vi "UHR-Fleezers Control (host) - 11.9.vi"() -> ()   [LabVIEW 2014] (continued)
        n1091 = xnode "Read/Write Control"("FPGA VI Reference In"=w1467, "error in"=w1468, "+ phase (APD 2 Gate)"=w1465) -> ("error out"=w1466:errorcluster)  [unwired: 1 out]
      }
      event "Phase Adj. (APD Acq)", "+ phase (APD Acq)", "- phase (APD Acq)": Value Change {
        n1092 = event-data() -> ()  [unwired: 7 out]
        n1093 = local read "Phase Adj. (APD Acq)"() -> (w1475:i16)
        n1094 = Negate(x=w1475) -> (-x=w1481:i16)
        n1095 = Select(t=w1481, s="+ phase (APD Acq)", f=w1475) -> (s? t:f=w1480:i16)
        n1096 = Or(x="+ phase (APD Acq)", y="- phase (APD Acq)") -> (x .or. y?=w1476:bool)
        n1097 = xnode "Read/Write Control"("FPGA VI Reference In"=w1483, "error in"=w1482, "Phase Count Adjustment (APD Acq)"=w1480) -> ("FPGA VI Reference Out"=w1478:T19, "error out"=w1479:errorcluster)
        n1098 = xnode "Read/Write Control"("FPGA VI Reference In"=w1478, "error in"=w1479, "+ phase (APD Acq)"=w1476) -> ("error out"=w1477:errorcluster)  [unwired: 1 out]
      }
      event "Phase adj. (GI)", "+ phase (GI)", "- phase (GI)": Value Change {
        n1099 = event-data() -> ()  [unwired: 7 out]
        n1100 = Negate(x="Phase adj. (GI)") -> (-x=w1492:i16)
        n1101 = Select(t=w1492, s="+ phase (GI)", f="Phase adj. (GI)") -> (s? t:f=w1491:i16)
        n1102 = Or(x="+ phase (GI)", y="- phase (GI)") -> (x .or. y?=w1487:bool)
        n1103 = xnode "Read/Write Control"("FPGA VI Reference In"=w1494, "error in"=w1493, "Phase count adjustment (GI)"=w1491) -> ("FPGA VI Reference Out"=w1489:T19, "error out"=w1490:errorcluster)
        n1104 = xnode "Read/Write Control"("FPGA VI Reference In"=w1489, "error in"=w1490, "+ phase (GI)"=w1487) -> ("error out"=w1488:errorcluster)  [unwired: 1 out]
      }
      event "Phase adj. (GI) 2", "+ phase (GI) 2", "- phase (GI) 2": Value Change {
        n1105 = event-data() -> ()  [unwired: 7 out]
        n1106 = Negate(x="Phase adj. (GI) 2") -> (-x=w1503:i16)
        n1107 = Select(t=w1503, s="+ phase (GI) 2", f="Phase adj. (GI) 2") -> (s? t:f=w1502:i16)
        n1108 = Or(x="+ phase (GI) 2", y="- phase (GI) 2") -> (x .or. y?=w1498:bool)
        n1109 = xnode "Read/Write Control"("FPGA VI Reference In"=w1505, "error in"=w1504, "Phase count adjustment (GI) 2"=w1502) -> ("FPGA VI Reference Out"=w1500:T19, "error out"=w1501:errorcluster)
        n1110 = xnode "Read/Write Control"("FPGA VI Reference In"=w1500, "error in"=w1501, "+ phase (GI) 2"=w1498) -> ("error out"=w1499:errorcluster)  [unwired: 1 out]
      }
      event "Phase adj. (Green FB)", "- phase (Green FB)", "+ phase (Green FB)": Value Change {
        n1111 = event-data() -> ()  [unwired: 7 out]
        n1112 = Negate(x="Phase adj. (Green FB)") -> (-x=w1514:i16)
        n1113 = Select(t=w1514, s="+ phase (Green FB)", f="Phase adj. (Green FB)") -> (s? t:f=w1513:i16)
        n1114 = Or(x="+ phase (Green FB)", y="- phase (Green FB)") -> (x .or. y?=w1509:bool)
        n1115 = xnode "Read/Write Control"("FPGA VI Reference In"=w1516, "error in"=w1515, "Phase count adjustment (Green FB)"=w1513) -> ("FPGA VI Reference Out"=w1511:T19, "error out"=w1512:errorcluster)
        n1116 = xnode "Read/Write Control"("FPGA VI Reference In"=w1511, "error in"=w1512, "+ phase (Green FB)"=w1509) -> ("error out"=w1510:errorcluster)  [unwired: 1 out]
      }
      event "Invert APD Gate", "APD Gate ON Count", "APD Gate OFF Count", "APD Gate", "APD Integration Time (s)", "APD 1 AO Mult.", "APD 2 AO Mult.", "On one out of X cycles": Value Change {
        n1117 = event-data() -> ()  [unwired: 7 out]
        n1118 = Add(x="GI Frequency, ON count", y="GI Frequency, OFF count") -> (x+y=w1520:u32)
        n1119 = Add(x="APD Gate ON Count", y="APD Gate OFF Count") -> (x+y=w1533:u32)
        n1120 = Multiply(x="On one out of X cycles", y=w1520) -> (x*y=w1517:u32)
        "Green FB Count" <- w1517
        n1121 = Subtract(x=w1517, y="GI Frequency, ON count") -> (x-y=w1518:u32)
        n1122 = Multiply(x=w1533, y="On one out of X cycles") -> (x*y=w1532:u32)
        n1123 = Subtract(x=w1532, y="APD Gate ON Count") -> (x-y=w1531:u32)
        n1124 = local read "DMA Update Period (s)"() -> (w1534:dbl)
        n1125 = Multiply(x="APD Integration Time (s)", y=40000000.0) -> (x*y=w1539:dbl)
        n1126 = Reciprocal(x="APD Integration Time (s)") -> (1/x=→"APD Acq Rate (Hz)":dbl)
        n1127 = To Unsigned Long Integer(number=w1539) -> (unsigned 32bit integer=w1523:u32)
        "APD Int. Count" <- w1523
        n1128 = xnode "Read/Write Control"("FPGA VI Reference In"=w1543, "error in"=w1542, "Invert APD Gate"="Invert APD Gate", "APD Gate ON Count"="APD Gate ON Count", "APD Gate OFF Count"=w1531, "APD Acq Rate Count"=w1523, "APD Gate Operating Mode"="APD Gate", "APD 1 AO scale factor"="APD 1 AO Mult.", "APD 2 AO scale factor"="APD 2 AO Mult.", "Green interlace ON count"="GI Frequency, ON count", "Green interlace OFF count"=w1518, "Green interlace ON count 2"="GI Frequency, ON count", "Green interlace OFF count 2"=w1518, "Green FB Count"=w1517) -> ("error out"=w1541:errorcluster)  [unwired: 1 out]
        n1129 = Divide(x=w1534, y="APD Integration Time (s)") -> (x/y=w1537:dbl)
        n1130 = Multiply(x=2.0, y=w1537) -> (x*y=w1536:dbl)
        n1131 = local write "APD Samples/FIFO Acq."(w1537) -> ()
        n1132 = local write "APD Elements/DMA read"(w1536) -> ()
      }
      event "Number of F/B Scans (AOD)", "Scan Speed (nm/s)", "Scan BD", "Initial D (MHz)", "Step Size (nm)", "Scan Range (nm)", "Wiggle amp 1 (units?)": Value Change {
        w1605 = 123.0  # AOM cal (nm/MHz)
        n1133 = event-data() -> ()  [unwired: 7 out]
        n1134 = local read "BD 1 Frequency 1 (MHz)"() -> (w1588:dbl)
        n1135 = local read "AOM X Cal (nm/MHz)"() -> (w1580:dbl)
        n1136 = local read "BD 2 Frequency 1 (MHz)"() -> (w1594:dbl)
        n1137 = local read "X RF Frequency Limits (MHz)"() -> (w1592:T16)
        n1138 = local read "Y RF Frequency Limits (MHz)"() -> (w1589:T16)
        n1139 = Negate(x="Scan Range (nm)") -> (-x=w1558:dbl)
        n1140 = Divide(x=w1558, y=w1580) -> (x/y=w1562:dbl)
        n1141 = Select(t=w1592, s="Scan BD", f=w1589) -> (s? t:f=w1591:T16)
        n1142 = Select(t=w1588, s="Scan BD", f=w1594) -> (s? t:f=w1593:dbl)
        n1143 = Unbundle By Name(w1591) -> ("Maximum"=w1600:dbl, "Minimum"=w1599:dbl)
        n1144 = Add(x=w1562, y=w1593) -> (x+y=w1597:dbl)
        n1145 = Divide(x=w1558, y="Step Size (nm)") -> (x/y=w1577:dbl)
        n1146 = Divide(x="Step Size (nm)", y=w1580) -> (x/y=w1586:dbl)
        n1147 = Absolute Value(x=w1577) -> (abs(x)=w1561:dbl)
        n1148 = Sign(1:w1558) -> (0:w1559:dbl)
        n1149 = In Range and Coerce(upper limit=w1600, x=w1597, lower limit=w1599) -> (coerced(x)=w1596:dbl, In Range?=w1598:bool)
        n1150 = To Unsigned Quad Integer(1:w1561) -> (0:w1576:u64)
        "Scan steps (AOD)" <- w1576
        n1151 = call "IR AOM freq to word.vi"("Frequency In (MHz)"=w1586) -> ("Frequency Word Out (double)"=w1583:dbl)
        n1152 = Multiply(x=w1559, y=w1583) -> (x*y=w1560:dbl)
        n1153 = Subtract(x=w1597, y=w1596) -> (x-y=w1595:dbl)
        n1154 = To Quad Integer(1:w1560) -> (0:w1582:i64)
        "Incr. int (AOD)" <- w1582
        n1155 = Subtract(x=w1562, y=w1595) -> (x-y=w1581:dbl)
        "Scan Range (MHz)" <- w1581
        n1156 = Select(t=w1562, s=w1598, f=w1581) -> (s? t:f=w1601:dbl)
        n1157 = Multiply(x=w1581, y=w1580) -> (x*y=w1579:dbl)
        n1158 = Decrement(x=w1576) -> (x-1=w1629:u64)
        n1159 = Negate(x=w1579) -> (-x=w1575:dbl)
        n1160 = local write "Scan Range (nm)"(w1575) -> ()
        n1161 = Divide(x=w1601, y=w1629) -> (x/y=w1585:dbl)
        "Scan Increment (MHz)" <- w1585
        n1162 = call "IR AOM freq to word.vi"("Frequency In (MHz)"=w1585) -> ("Frequency Word Out (double)"=w1584:dbl)
        n1163 = Divide(x="Step Size (nm)", y="Scan Speed (nm/s)") -> (x/y=w1572:dbl)
        n1164 = To Quad Integer(1:w1584) -> ()  [unwired: 1 out]
        n1165 = local read "Number Interlace Sets"() -> (w1556:u8)
        n1166 = local read "AI Count (ticks)"() -> (w1557:u32)
        n1167 = local read "Total Counts (ticks)"() -> (w1555:u32)
        n1168 = local read "# Samples/trap"() -> (w1587:u32)
        n1169 = Multiply(x=w1557, y=w1556) -> (x*y=w1554:u32)
        n1170 = Divide(x=w1555, y=w1554) -> (x/y=w1553:dbl)
        n1171 = Select(t=w1588, s="Scan BD", f=w1594) -> (s? t:f=w1626:dbl)
        "Initial freq. (MHz)" <- w1626
        n1172 = Add(x=w1601, y=w1626) -> (x+y=→"Final freq. (MHz)":dbl)
        n1173 = Divide(x=w1555, y=40000000.0) -> (x/y=w1571:dbl)
        n1174 = Divide(x=w1572, y=w1571) -> (x/y=w1570:dbl)
        n1175 = To Unsigned Quad Integer(1:w1570) -> (0:w1545:u64)
        n1176 = Quotient & Remainder(x=w1545, y=u64 2) -> (x-y*floor(x/y)=w1549:u64)  [unwired: 1 out]
        n1177 = Equal?(x=w1549, y=u64 0) -> (x = y?=w1547:bool)
        n1178 = Decrement(x=w1545) -> (x-1=w1546:u64)
        n1179 = Select(t=w1545, s=w1547, f=w1546) -> (s? t:f=w1544:u64)
        "Cycles/step (AOD)" <- w1544
        n1180 = xnode "Read/Write Control"("FPGA VI Reference In"=w1637, "error in"=w1636, "Scan steps"=w1576, "Number of scans"="Number of F/B Scans (AOD)", "Cycles per step"=w1544, "Scan freq.  increment"=w1582, "Scan BD"="Scan BD") -> ("error out"=w1635:errorcluster)  [unwired: 1 out]
        n1181 = Multiply(x=w1576, y=w1544) -> (x*y=w1630:u64)
        n1182 = Multiply(x=w1630, y=u64 2) -> (x*y=w1552:u64)
        n1183 = Multiply(x=w1553, y=w1552) -> (x*y=w1551:dbl)
        "Data points/scan (f/b)" <- w1551
        n1184 = Multiply(x=w1551, y="Number of F/B Scans (AOD)") -> (x*y=w1633:dbl)
        "Data points/scans" <- w1633
        n1185 = Divide(x=w1633, y=w1587) -> (x/y=→"N sets should be saved":dbl)
        n1186 = Multiply(x=w1630, y=w1571) -> (x*y=w1569:dbl)
        "Time/Scan (s) (AOD)" <- w1569
        n1187 = Select(t=w1601, s="Scan BD", f=0.0) -> (s? t:f=w1627:dbl)
        n1188 = Select(t=0.0, s="Scan BD", f=w1601) -> (s? t:f=w1623:dbl)
        n1189 = local read "BD 2 Frequency 2 (MHz)"() -> (w1619:dbl)
        n1190 = local read "BD 1 Frequency 2 (MHz)"() -> (w1622:dbl)
        n1191 = Add(x=w1623, y=w1594) -> (x+y=w1620:dbl)
        n1192 = Add(x=w1588, y=w1627) -> (x+y=w1621:dbl)
        n1193 = Multiply(x=w1569, y=2.0) -> (x*y=w1568:dbl)
        n1194 = Multiply(x=w1568, y="Number of F/B Scans (AOD)") -> (x*y=w1565:dbl)
        n1195 = Divide(x=w1565, y=60.0) -> (x/y=→"Time to Finish All (min)":dbl)
        n1196 = Add(x="Trap 2 Bead Size (nm)", y="Trap 1 Bead Size (nm)") -> (x+y=w1609:dbl)
        n1197 = Divide(x=w1609, y=2.0) -> (x/y=w1603:dbl)
        n1198 = Subtract(x=w1620, y=w1619) -> (x-y=w1617:dbl)
        n1199 = Subtract(x=w1621, y=w1622) -> (x-y=w1618:dbl)
        n1200 = local read "Initial D (MHz)"() -> (w1606:dbl)
        n1201 = Square(x=w1617) -> (x^2=w1616:dbl)
        n1202 = Square(x=w1618) -> (x^2=w1615:dbl)
        n1203 = Add(x=w1615, y=w1616) -> (x+y=w1614:dbl)
        n1204 = Square Root(x=w1614) -> (sqrt(x)=w1613:dbl)
        "Final D (MHz)" <- w1613
        n1205 = Multiply(x=w1605, y=w1613) -> (x*y=w1612:dbl)
        n1206 = Multiply(x=w1606, y=w1605) -> (x*y=w1604:dbl)
        n1207 = Subtract(x=w1604, y=w1603) -> (x-y=→"Initial sep (nm)":dbl)
        n1208 = Subtract(x=w1612, y=w1603) -> (x-y=→"Final sep (nm)":dbl)
      }
      event "Freq or Amp switch first", "Swap F1 and F2", "Freq switch delay", "Amp switch delay": Value Change {
        n1209 = event-data() -> ()  [unwired: 7 out]
        n1210 = local read "Freq or Amp switch first"() -> (w1638:bool)
        n1211 = local read "Amp switch delay"() -> (w1639:u16)
        n1212 = local read "Freq switch delay"() -> (w1641:u16)
        n1213 = local read "Swap F1 and F2"() -> (w1640:bool)
        n1214 = xnode "Read/Write Control"("FPGA VI Reference In"=w1644, "error in"=w1643, "Freq switch delay"=w1641, "Swap F1 and F2"=w1640, "Amp switch delay"=w1639, "Freq or Amp switch first"=w1638) -> ("error out"=w1642:errorcluster)  [unwired: 1 out]
      }
      event "Scan steps (MCL)", "Number of scans (MCL)", "Scan Range (V)\n(of steps)", "2D or 1D Scan", "N APD Samp/step", "Fast Scan Dir", "Continuous MCL Scanning", "Scan lines (y)": Value Change {
        w1646 = 32767.0 ("y")
        n1215 = event-data() -> ()  [unwired: 7 out]
        n1216 = Select(t="Scan lines (y)", s="2D or 1D Scan", f="Number of scans (MCL)") -> (s? t:f=w1651:u64)
        n1217 = Decrement(x="Scan steps (MCL)") -> (x-1=w1667:u64)
        n1218 = Divide(x="Scan Range (V)\n(of steps)", y=w1667) -> (x/y=w1666:dbl)
        "Desired Scan Incr (V)" <- w1666
        n1219 = local read "APD Integration Time (s)"() -> (w1659:dbl)
        n1220 = Multiply(x=w1666, y=w1646) -> (x*y=w1675:dbl)
        n1221 = Divide(x=w1675, y=10.0) -> (x/y=w1665:dbl)
        "Desired incr (int)" <- w1665
        n1222 = local read "Update Count (MCL)"() -> (w1671:u32)
        n1223 = Round Toward -Infinity(1:w1665) -> (0:w1674:dbl)
        n1224 = To Word Integer(number=w1674) -> (16bit integer=w1649:i16)
        "Actual Incr. int (MCL)" <- w1649
        n1225 = Multiply(x=w1659, y=40000000.0) -> (x*y=w1672:dbl)
        n1226 = Divide(x=w1672, y=w1671) -> (x/y=w1670:dbl)
        n1227 = Multiply(x=i16 10, y=w1649) -> (x*y=w1647:i16)
        n1228 = Multiply(x="N APD Samp/step", y=w1670) -> (x*y=w1669:dbl)
        "Cycles/step (MCL)" <- w1669
        n1229 = Divide(x=w1647, y=w1646) -> (x/y=→"Actual MCL Inc (V)":dbl)
        n1230 = Multiply(x="N APD Samp/step", y="Scan steps (MCL)") -> (x*y=w1661:dbl)
        n1231 = local read "APD Samples/FIFO Acq."() -> (w1658:dbl)
        n1232 = Multiply(x=w1661, y=u64 2) -> (x*y=w1660:dbl)
        "Data points/scan (f+b)" <- w1660
        n1233 = Multiply(x=w1660, y=w1651) -> (x*y=w1678:dbl)
        "Data points/scans (MCL)" <- w1678
        n1234 = Multiply(x=w1659, y=w1660) -> (x*y=w1652:dbl)
        "Time/f+b scan (s) (MCL)" <- w1652
        n1235 = Divide(x=w1678, y=w1658) -> (x/y=→"N sets should be saved (MCL)":dbl)
        n1236 = Multiply(x=w1652, y=w1651) -> (x*y=→"Total Time (s)":dbl)
        n1237 = Not(x="Fast Scan Dir") -> (.not. x?=w1656:bool)
        n1238 = xnode "Read/Write Control"("FPGA VI Reference In"=w1682, "error in"=w1681, "Scan steps (MCL)"="Scan steps (MCL)", "Number of scans (MCL)"=w1651, "Cycles per step (MCL)"=w1669, "Scan freq.  increment (MCL)"=w1649, "1D or 2D Scan?"="2D or 1D Scan", "MCL Scan Axis"=w1656, "Cont. Scan (MCL)"="Continuous MCL Scanning") -> ("error out"=w1680:errorcluster)  [unwired: 1 out]
      }
      event "Read Cal": Value Change {
        w1684 = 1000.0 ("y")
        n1239 = event-data() -> ()  [unwired: 7 out]
        n1240 = local read "Save file name"() -> (w1709:path)
        n1241 = local write "Read Cal"(FALSE ("Read Cal")) -> ()
        n1242 = Strip Path(path=w1709) -> (stripped path=w1708:path)  [unwired: 1 out]
        n1243 = Path To String(path=w1708) -> (string=w1707:string)
        n1244 = Concatenate Strings(w1707, "\\current.cal" ("string")) -> (w1705:string)
        n1245 = String To Path(string=w1705) -> (path=w1704:path)
        n1246 = Open/Create/Replace File(file path (use dialog)=w1704, operation (0:open)=T25."open", access (0:read/write)=enum16{"read/write", "read-only", "write-only"}."read-only") -> (refnum out=w1712:refnum<file>, error out=w1698:errorcluster)  [unwired: 1 in, 3 out]
        n1247 = Deny Access(4:w1698, 7:w1712) -> (0:w1697:errorcluster, 3:w1703:refnum<file>)  [unwired: 1 out]
        n1248 = Read from Binary File(5:0.0, 8:w1697, 9:T24."big-endian, network order" ("byte order (0:big-endian, network order)"), 10:-1 ("count (1)"), 11:w1703) -> (0:w1696:errorcluster, 2:w1694:dbl[], 3:w1699:refnum<file>)  [unwired: 2 out]
        n1249 = Array To Cluster(array=w1694) -> (cluster=w1693:T27)
        n1250 = Unbundle(w1693) -> ("[0]"=w1692:dbl, "[1]"=w1691:dbl, "[2]"=w1690:dbl, "[3]"=w1689:dbl, "[4]"=w1688:dbl, "[5]"=w1687:dbl)
        n1251 = Close File(refnum=w1699, error in=w1696) -> (error out=→"Read cal error":errorcluster)  [unwired: 1 out]
        n1252 = Multiply(x=w1687, y=w1684) -> (x*y=w1685:dbl)
        n1253 = local write "T2 k_x (pN/nm)"(w1689) -> ()
        n1254 = local write "T1 k_x (pN/nm)"(w1690) -> ()
        n1255 = local write "T1 a_x (nm/V)"(w1692) -> ()
        n1256 = local write "T2 a_x (nm/V)"(w1691) -> ()
        n1257 = Multiply(x=w1688, y=w1684) -> (x*y=w1686:dbl)
        n1258 = local write "T1 offset_x (mV)"(w1686) -> ()
        n1259 = local write "T2 offset_x (mV)"(w1685) -> ()
      }
      event "Read FX file": Value Change {
        n1260 = event-data() -> ()  [unwired: 7 out]
        n1261 = local write "Read FX file"(FALSE ("Read residual")) -> ()
        n1262 = local read "Save file name"() -> (w1737:path)
        n1263 = Strip Path(path=w1737) -> (stripped path=w1736:path)  [unwired: 1 out]
        n1264 = Path To String(path=w1736) -> (string=w1735:string)
        n1265 = Concatenate Strings(w1735, "\\current.cal" ("string")) -> (w1733:string)
        n1266 = String To Path(string=w1733) -> (path=w1732:path)
        n1267 = Open/Create/Replace File(file path (use dialog)=w1732, operation (0:open)=T25."open", access (0:read/write)=enum16{"read/write", "read-only", "write-only"}."read-only") -> (refnum out=w1729:refnum<file>, error out=w1726:errorcluster)  [unwired: 3 in, 1 out]
        n1268 = Deny Access(4:w1726, 7:w1729) -> (0:w1725:errorcluster, 3:w1728:refnum<file>)  [unwired: 1 in]
        n1269 = Read from Binary File(5:0.0, 8:w1725, 9:T24."big-endian, network order" ("byte order (0:big-endian, network order)"), 10:-1 ("count"), 11:w1728) -> (0:w1721:errorcluster, 2:w1715:dbl[], 3:w1722:refnum<file>)  [unwired: 1 in, 1 out]
        n1270 = Index Array(array=w1715, index=6) -> (element=→"Bad fit error":dbl)
        n1271 = Index Array(array=w1715, index=7) -> (element=→"Fit offset":dbl)
        n1272 = Index Array(array=w1715, index=8) -> (element=→"Hyst. error":dbl)
        n1273 = Close File(refnum=w1722, error in=w1721) -> ()  [unwired: 2 out]
      }
      event "Abort MCL Scan": Value Change {
        n1274 = event-data() -> ()  [unwired: 7 out]
        n1275 = local write "MCL Scanning"(FALSE ("MCL Scanning")) -> ()
        n1276 = xnode "Read/Write Control"("FPGA VI Reference In"=w1742, "error in"=w1741, "Abort scan (MCL)"="Abort MCL Scan") -> ("error out"=w1740:errorcluster)  [unwired: 1 out]
      }
      event "Update Count (MCL)": Value Change {
        n1277 = event-data() -> ()  [unwired: 7 out]
        n1278 = xnode "Read/Write Control"("FPGA VI Reference In"=w1746, "error in"=w1745, "MCL count"="Update Count (MCL)") -> ("error out"=w1744:errorcluster)  [unwired: 1 out]
      }
      event "Phase adjust (MCL)", "+ phase (MCL)", "- phase (MCL)": Value Change {
        n1279 = event-data() -> ()  [unwired: 7 out]
        n1280 = Negate(x="Phase adjust (MCL)") -> (-x=w1755:i16)
        n1281 = Select(t=w1755, s="- phase (MCL)", f="Phase adjust (MCL)") -> (s? t:f=w1753:i16)
        n1282 = Or(x="- phase (MCL)", y="+ phase (MCL)") -> (x .or. y?=w1748:bool)
        n1283 = xnode "Read/Write Control"("FPGA VI Reference In"=w1757, "error in"=w1756, "Phase count adjustment (MCL)"=w1753) -> ("FPGA VI Reference Out"=w1749:T19, "error out"=w1750:errorcluster)
        n1284 = xnode "Read/Write Control"("FPGA VI Reference In"=w1749, "error in"=w1750, "+ phase (MCL)"=w1748) -> ("error out"=w1747:errorcluster)  [unwired: 1 out]
      }
      event "Abort AOD Scan": Value Change {
        n1285 = event-data() -> ()  [unwired: 7 out]
        n1286 = xnode "Read/Write Control"("FPGA VI Reference In"=w1761, "error in"=w1760, "Abort scan"="Abort AOD Scan") -> ("error out"=w1759:errorcluster)  [unwired: 1 out]
      }
      event "Continuous AOD Scanning": Value Change {
        n1287 = event-data() -> ()  [unwired: 7 out]
        n1288 = xnode "Read/Write Control"("FPGA VI Reference In"=w1765, "error in"=w1764, "Cont. Scan"="Continuous AOD Scanning") -> ("error out"=w1763:errorcluster)  [unwired: 1 out]
      }
      event "Index": Value Change {
        n1289 = event-data() -> ()  [unwired: 7 out]
        n1290 = call "Create new save file.vi"("Insert"="", "Ext"=".dat" ("string"), "Index In"="Index") -> ("Path Out"=→"Save file name":path, "Index Out"=w1766:dbl)
        "Save index" <- w1766
        n1291 = local write "Index"(w1766) -> ()
      }
      event "AO1", "AO2": Value Change {
        w1781 = 10.0 ("y")
        w1780 = 32767.0 ("y")
        n1292 = event-data() -> ()  [unwired: 7 out]
        n1293 = local read "AO2"() -> (w1779:dbl)
        n1294 = local read "AO1"() -> (w1776:dbl)
        n1295 = Multiply(x=w1776, y=w1780) -> (x*y=w1775:dbl)
        n1296 = Multiply(x=w1779, y=w1780) -> (x*y=w1778:dbl)
        n1297 = Divide(x=w1775, y=w1781) -> (x/y=w1774:dbl)
        n1298 = Divide(x=w1778, y=w1781) -> (x/y=w1777:dbl)
        n1299 = To Word Integer(number=w1774) -> (16bit integer=w1782:i16)
        n1300 = To Word Integer(number=w1777) -> (16bit integer=w1783:i16)
        n1301 = xnode "Read/Write Control"("FPGA VI Reference In"=w1773, "error in"=w1772, "AO1"=w1782, "AO2"=w1783) -> ("error out"=w1771:errorcluster)  [unwired: 1 out]
      }
      event "Inject Pump 1": Value Change {
        n1302 = event-data() -> ()  [unwired: 7 out]
        n1303 = local read "Use Harvard pumps\nfor beads (else Chemyx)"() -> (w1785:bool)
        n1304 = case shown="True" w1785 {
          tunnel: "Inject Pump 1" -> [w1789 w1827]
          tunnel: w1784 -> [_ w1828]
          frame False {
            n1305 = local read "Pump write delay (ms)"() -> (w1788:dbl)
            n1306 = local read "Chemyx Syringe Pump Serial Port"() -> (w1787:refnum<visa-resource-name>)
            n1307 = case shown="True" w1789 {
              tunnel: w1788 -> [w1795 w1809]
              tunnel: w1787 -> [w1792 w1808]
              frame False {
                n1308 = flat-sequence {
                  tunnel: w1792 -> [w1796]
                  tunnel: [w1796] -> w1793
                  tunnel: w1795 -> [_]
                  tunnel: [w1799] -> w1794
                  tunnel: w1793 -> [w1799]
                  tunnel: w1794 -> [w1800]
                  tunnel: [w1800] -> w1790
                  tunnel: [w1802] -> w1791
                  tunnel: w1790 -> [w1802]
                  tunnel: w1791 -> [w1804]
                  frame #0 {
                    n1309 = call "Write to pump.vi"("string"="enter pump1", "VISA resource name"=w1796) -> ()  [unwired: 1 out]
                  }
                  frame #1 {
                    n1310 = Wait (ms)(milliseconds to wait="Pump pause delay (ms)") -> ()  [unwired: 1 out]
                  }
                  frame #2 {
                    n1311 = call "Write to pump.vi"("string"="stop", "VISA resource name"=w1800) -> ()  [unwired: 1 out]
                  }
                  frame #3 {
                    n1312 = Wait (ms)(milliseconds to wait=u32 500) -> ()  [unwired: 1 out]
                  }
                  frame #4 {
                    n1313 = call "Write to pump.vi"("string"="stop", "VISA resource name"=w1804) -> ()  [unwired: 1 out]
                  }
                }
              }
              frame True {
                n1314 = flat-sequence {
                  tunnel: w1808 -> [w1818]
                  tunnel: w1809 -> [w1813]
                  tunnel: w1809 -> [w1820]
                  tunnel: w1808 -> [w1821]
                  tunnel: [w1821] -> w1806
                  tunnel: [w1823] -> w1807
                  tunnel: w1806 -> [w1823]
                  tunnel: w1807 -> [w1825]
                  frame #0 {
                    n1315 = local read "All Pump Parameters"() -> (w1812:T5)
                    n1316 = Unbundle By Name(w1812) -> ("Pump 1"=w1819:T28)
                    n1317 = call "Set pump parameters.vi"("Pump write delay (ms)"=w1813, "Volume (uL)"="Ch 1 Inject Volume (uL)", "Rate (uL/h)"="Ch 1 Inject Rate (ul/h)", "Units"=4.0, "Pump #"=1.0, "Pump Parameters In"=w1819, "VISA resource name"=w1818) -> ("Pump Parameters Out"=w1811:T28)  [unwired: 3 in]
                    n1318 = Bundle By Name(cluster=w1812, "Pump 1"=w1811) -> (w1810:T5)
                    n1319 = local write "All Pump Parameters"(w1810) -> ()
                  }
                  frame #1 {
                    n1320 = Wait (ms)(milliseconds to wait=w1820) -> ()  [unwired: 1 out]
                  }
                  frame #2 {
                    n1321 = call "Write to pump.vi"("string"="start", "VISA resource name"=w1821) -> ()  [unwired: 1 out]
                  }
                  frame #3 {
                    n1322 = Wait (ms)(milliseconds to wait=u32 500) -> ()  [unwired: 1 out]
                  }
                  frame #4 {
                    n1323 = call "Write to pump.vi"("string"="start", "VISA resource name"=w1825) -> ()  [unwired: 1 out]
                  }
                }
              }
            }
          }
          frame True {
            n1324 = case shown="True" w1827 {
              tunnel: w1828 -> [w1829 w1839]
              frame False {
                n1325 = flat-sequence {
                  tunnel: w1829 -> [w1831]
                  frame #0 {
                    n1326 = local write "Flushing P1"(FALSE ("Flushing P1")) -> ()
                    n1327 = Concatenate Strings("stop" ("string"), "\r") -> (w1833:string)
                    n1328 = VISA Write(VISA resource name=w1831, write buffer=w1833) -> ()  [unwired: 1 in, 3 out]
                  }
                  frame #1 {
                    n1329 = property on="Clear Volume P1" class="Bool (strict)"("Val(Sgnl)"=TRUE ("Value (Signaling)")) -> ()  [unwired: 2 in, 2 out]
                  }
                }
              }
              frame True {
                n1330 = local read "Normal Flow Rate (ul/h) P1"() -> (w1837:dbl)
                n1331 = Number To Decimal String(number=w1837) -> (decimal integer string=w1843:string)  [unwired: 1 in]
                n1332 = Concatenate Strings("irate  " ("string"), w1843, " u/h" ("string"), "\r") -> (w1841:string)
                n1333 = VISA Write(VISA resource name=w1839, write buffer=w1841) -> (VISA resource name out=w1838:refnum<visa-resource-name>)  [unwired: 1 in, 2 out]
                n1334 = Concatenate Strings("irun" ("string"), "\r") -> (w1845:string)
                n1335 = VISA Write(VISA resource name=w1838, write buffer=w1845) -> ()  [unwired: 1 in, 3 out]
              }
            }
          }
        }
      }
      event "Inject Pump 3": Value Change {
        n1336 = event-data() -> ()  [unwired: 7 out]
        n1337 = local read "Use Harvard pumps\nfor beads (else Chemyx)"() -> (w1848:bool)
        n1338 = case shown="True" w1848 {
          tunnel: "Inject Pump 3" -> [w1852 w1891]
          tunnel: w1847 -> [_ w1890]
          frame False {
            n1339 = local read "Pump write delay (ms)"() -> (w1851:dbl)
            n1340 = case shown="True" w1852 {
              tunnel: w1851 -> [w1858 w1872]
              tunnel: "Chemyx Syringe Pump Serial Port" -> [w1855 w1871]
              frame False {
                n1341 = flat-sequence {
                  tunnel: w1855 -> [w1859]
                  tunnel: [w1859] -> w1856
                  tunnel: w1858 -> [_]
                  tunnel: [w1862] -> w1857
                  tunnel: w1856 -> [w1862]
                  tunnel: w1857 -> [w1863]
                  tunnel: [w1863] -> w1853
                  tunnel: [w1865] -> w1854
                  tunnel: w1853 -> [w1865]
                  tunnel: w1854 -> [w1867]
                  frame #0 {
                    n1342 = call "Write to pump.vi"("string"="enter pump3", "VISA resource name"=w1859) -> ()  [unwired: 1 out]
                  }
                  frame #1 {
                    n1343 = local read "Pump pause delay (ms)"() -> (w1861:u32)
                    n1344 = Wait (ms)(milliseconds to wait=w1861) -> ()  [unwired: 1 out]
                  }
                  frame #2 {
                    n1345 = call "Write to pump.vi"("string"="stop", "VISA resource name"=w1863) -> ()  [unwired: 1 out]
                  }
                  frame #3 {
                    n1346 = Wait (ms)(milliseconds to wait=u32 0) -> ()  [unwired: 1 out]
                  }
                  frame #4 {
                    n1347 = call "Write to pump.vi"("string"="stop", "VISA resource name"=w1867) -> ()  [unwired: 1 out]
                  }
                }
              }
              frame True {
                n1348 = flat-sequence {
                  tunnel: w1871 -> [w1881]
                  tunnel: w1872 -> [w1876]
                  tunnel: w1872 -> [w1883]
                  tunnel: w1871 -> [w1884]
                  tunnel: [w1884] -> w1870
                  tunnel: [w1887] -> w1869
                  tunnel: w1870 -> [w1887]
                  tunnel: w1869 -> [w1888]
                  frame #0 {
                    n1349 = local read "All Pump Parameters"() -> (w1875:T5)
                    n1350 = Unbundle By Name(w1875) -> ("Pump 3"=w1882:T28)
                    n1351 = call "Set pump parameters.vi"("Pump write delay (ms)"=w1876, "Volume (uL)"="Ch 3 Inject Volume (uL)", "Rate (uL/h)"="Ch 3 Inject Rate (ul/h)", "Units"=4.0, "Pump #"=3.0, "Pump Parameters In"=w1882, "VISA resource name"=w1881) -> ("Pump Parameters Out"=w1874:T28)  [unwired: 3 in]
                    n1352 = Bundle By Name(cluster=w1875, "Pump 3"=w1874) -> (w1873:T5)
                    n1353 = local write "All Pump Parameters"(w1873) -> ()
                  }
                  frame #1 {
                    n1354 = Wait (ms)(milliseconds to wait=w1883) -> ()  [unwired: 1 out]
                  }
                  frame #2 {
                    n1355 = call "Write to pump.vi"("string"="start", "VISA resource name"=w1884) -> ()  [unwired: 1 out]
                  }
                  frame #3 {
                    n1356 = Wait (ms)(milliseconds to wait=u32 500) -> ()  [unwired: 1 out]
                  }
                  frame #4 {
                    n1357 = call "Write to pump.vi"("string"="start", "VISA resource name"=w1888) -> ()  [unwired: 1 out]
                  }
                }
              }
            }
          }
          frame True {
            n1358 = case shown="True" w1891 {
              tunnel: w1890 -> [w1892 w1899]
              frame False {
                n1359 = flat-sequence {
                  tunnel: w1892 -> [w1894]
                  frame #0 {
                    n1360 = local write "Flushing P3"(FALSE ("Flushing P3")) -> ()
                    n1361 = Concatenate Strings("stop" ("string"), "\r") -> (w1896:string)
                    n1362 = VISA Write(VISA resource name=w1894, write buffer=w1896) -> ()  [unwired: 1 in, 3 out]
                  }
                  frame #1 {
                    n1363 = property on="Clear Volume P3" class="Bool (strict)"("Val(Sgnl)"=TRUE ("Value (Signaling)")) -> ()  [unwired: 2 in, 2 out]
                  }
                }
              }
              frame True {
                n1364 = local read "Normal Flow Rate (ul/h) P3"() -> (w1900:dbl)
                n1365 = Number To Decimal String(number=w1900) -> (decimal integer string=w1906:string)  [unwired: 1 in]
                n1366 = Concatenate Strings("irate  " ("string"), w1906, " u/h" ("string"), "\r") -> (w1904:string)
                n1367 = VISA Write(VISA resource name=w1899, write buffer=w1904) -> (VISA resource name out=w1902:refnum<visa-resource-name>)  [unwired: 1 in, 2 out]
                n1368 = Concatenate Strings("irun" ("string"), "\r") -> (w1908:string)
                n1369 = VISA Write(VISA resource name=w1902, write buffer=w1908) -> ()  [unwired: 1 in, 3 out]
              }
            }
          }
        }
      }
      event "Inject Pump 2": Value Change {
        n1370 = event-data() -> ()  [unwired: 7 out]
        n1371 = local read "Pump write delay (ms)"() -> (w1912:dbl)
        n1372 = local read "Chemyx Syringe Pump Serial Port"() -> (w1910:refnum<visa-resource-name>)
        n1373 = flat-sequence {
          tunnel: w1910 -> [w1925]
          tunnel: w1912 -> [w1921]
          tunnel: "Inject Pump 2" -> [_]
          tunnel: w1912 -> [w1927]
          tunnel: w1910 -> [w1928]
          frame #0 {
            n1374 = local read "All Pump Parameters"() -> (w1920:T5)
            n1375 = Multiply(x=60.0, y="Flush Center Ch Rate (ul/m)") -> (x*y=w1917:dbl)
            n1376 = Unbundle By Name(w1920) -> ("Pump 2"=w1926:T28)
            n1377 = call "Set pump parameters.vi"("Pump write delay (ms)"=w1921, "Volume (uL)"="Flush Center Ch Volume (uL)", "Rate (uL/h)"=w1917, "Units"=3.0, "Pump #"=2.0, "Pump Parameters In"=w1926, "VISA resource name"=w1925) -> ("Pump Parameters Out"=w1919:T28)  [unwired: 3 in]
            n1378 = Bundle By Name(cluster=w1920, "Pump 2"=w1919) -> (w1918:T5)
            n1379 = Add(x="Flush Center Ch Volume (uL)", y="Total Volume\nFlushed (uL)") -> (x+y=w1914:dbl)
            n1380 = local write "All Pump Parameters"(w1918) -> ()
            n1381 = local write "Total Volume\nFlushed (uL)"(w1914) -> ()
          }
          frame #1 {
            n1382 = Wait (ms)(milliseconds to wait=w1927) -> ()  [unwired: 1 out]
          }
          frame #2 {
            n1383 = call "Write to pump.vi"("string"="start", "VISA resource name"=w1928) -> ()  [unwired: 1 out]
          }
        }
      }
      event "Sample Channel\nFlow": Value Change {
        n1384 = event-data() -> ()  [unwired: 7 out]
        n1385 = case shown="True" "Sample Channel\nFlow" {
          tunnel: w1931 -> [w1932 w1938]
          frame False {
            n1386 = flat-sequence {
              tunnel: w1932 -> [w1934]
              frame #0 {
                n1387 = local write "Flushing samp"(FALSE ("Flushing samp")) -> ()
                n1388 = Concatenate Strings("stop" ("string"), "\r") -> (w1937:string)
                n1389 = VISA Write(VISA resource name=w1934, write buffer=w1937) -> ()  [unwired: 1 in, 3 out]
              }
            }
          }
          frame True {
            n1390 = local read "Normal Flow rate (mL/h)"() -> (w1948:dbl)
            n1391 = Number To Decimal String(number=w1948) -> (decimal integer string=w1947:string)  [unwired: 1 in]
            n1392 = Concatenate Strings("irate " ("string"), w1947, " u/h" ("string"), "\r") -> (w1943:string)
            n1393 = VISA Write(VISA resource name=w1938, write buffer=w1943) -> (VISA resource name out=w1942:refnum<visa-resource-name>)  [unwired: 1 in, 2 out]
            n1394 = Concatenate Strings("irun" ("string"), "\r") -> (w1939:string)
            n1395 = VISA Write(VISA resource name=w1942, write buffer=w1939) -> ()  [unwired: 1 in, 3 out]
          }
        }
      }
      event "Start Flow": Value Change {
        n1396 = event-data() -> ()  [unwired: 7 out]
        n1397 = local write "Sample Channel\nFlow"(TRUE ("Sample Channel\nFlow")) -> ()
        n1398 = local write "Start Flow"(FALSE ("Start Flow")) -> ()
        n1399 = Concatenate Strings("irun" ("string"), "\r") -> (w1953:string)
        n1400 = VISA Write(VISA resource name=w1949, write buffer=w1953) -> ()  [unwired: 1 in, 3 out]
      }
      event "Stop Flow": Value Change {
        w1955 = FALSE ("Stop Flow")
        n1401 = event-data() -> ()  [unwired: 7 out]
        n1402 = local write "Stop Flow"(w1955) -> ()
        n1403 = local write "Sample Channel\nFlow"(w1955) -> ()
        n1404 = Concatenate Strings("stop" ("string"), "\r") -> (w1958:string)
        n1405 = VISA Write(VISA resource name=w1956, write buffer=w1958) -> ()  [unwired: 1 in, 3 out]
      }
      event "Normal Flow rate (mL/h)": Value Change {
        n1406 = event-data() -> ()  [unwired: 7 out]
        n1407 = Number To Decimal String(number="Normal Flow rate (mL/h)") -> (decimal integer string=w1965:string)  [unwired: 1 in]
        n1408 = Concatenate Strings("irate  " ("string"), w1965, " u/h" ("string"), "\r") -> (w1964:string)
        n1409 = VISA Write(VISA resource name=w1961, write buffer=w1964) -> ()  [unwired: 1 in, 3 out]
      }
      event "Flush Sample": Value Change {
        n1410 = event-data() -> ()  [unwired: 7 out]
        n1411 = flat-sequence {
          tunnel: w1967 -> [w1995]
          frame #0 {
            # "set parameters (rate, volume) for flush, clear volume"
            n1412 = Number To Decimal String(number="Flush rate (mL/m)") -> (decimal integer string=w1991:string)  [unwired: 1 in]
            n1413 = local write "Sample Channel\nFlow"(TRUE ("Sample Channel\nFlow")) -> ()
            n1414 = Concatenate Strings("irate  " ("string"), w1991, " u/m" ("string"), "\r") -> (w1993:string)
            n1415 = VISA Write(VISA resource name=w1995, write buffer=w1993) -> (VISA resource name out=w1989:refnum<visa-resource-name>)  [unwired: 1 in, 2 out]
            n1416 = Number To Decimal String(number="Flush volume (mL)") -> (decimal integer string=w1980:string)  [unwired: 1 in]
            n1417 = Reciprocal(x="Flush rate (mL/m)") -> (1/x=w1974:dbl)
            n1418 = Concatenate Strings("tvolume  " ("string"), w1980, " u" ("string"), "\r") -> (w1978:string)
            n1419 = Multiply(x=w1974, y="Flush volume (mL)") -> (x*y=w1972:dbl)
            n1420 = VISA Write(VISA resource name=w1989, write buffer=w1978) -> (VISA resource name out=w1977:refnum<visa-resource-name>)  [unwired: 1 in, 2 out]
            n1421 = Multiply(x=w1972, y=60.0) -> (x*y=→"Samp Flush Time (s)":dbl)
            n1422 = Concatenate Strings("cvolume" ("string"), "\r") -> (w1976:string)
            n1423 = VISA Write(VISA resource name=w1977, write buffer=w1976) -> (VISA resource name out=w1987:refnum<visa-resource-name>)  [unwired: 1 in, 2 out]
            n1424 = Concatenate Strings("irun" ("string"), "\r") -> (w1985:string)
            n1425 = VISA Write(VISA resource name=w1987, write buffer=w1985) -> ()  [unwired: 1 in, 3 out]
          }
          frame #1 {
            "Flushing samp" <- TRUE ("Boolean")
          }
        }
      }
      event "Flush Pump 3": Value Change {
        n1426 = event-data() -> ()  [unwired: 7 out]
        n1427 = flat-sequence {
          tunnel: w1997 -> [w2000]
          frame #0 {
            # "set paramaters (rate, volume) for flush, clear volume"
            n1428 = Number To Decimal String(number="Flush rate (uL/m) P3") -> (decimal integer string=w2022:string)  [unwired: 1 in]
            n1429 = local write "Inject Pump 3"(TRUE ("Inject Pump 3")) -> ()
            n1430 = Concatenate Strings("irate  " ("string"), w2022, " u/m" ("string"), "\r") -> (w2024:string)
            n1431 = VISA Write(VISA resource name=w2000, write buffer=w2024) -> (VISA resource name out=w2020:refnum<visa-resource-name>)  [unwired: 1 in, 2 out]
            n1432 = Reciprocal(x="Flush rate (uL/m) P3") -> (1/x=w2004:dbl)
            n1433 = Number To Decimal String(number="Volume (uL) P3") -> (decimal integer string=w2011:string)  [unwired: 1 in]
            n1434 = Multiply(x="Volume (uL) P3", y=w2004) -> (x*y=w2003:dbl)
            n1435 = Concatenate Strings("tvolume  " ("string"), w2011, " u" ("string"), "\r") -> (w2009:string)
            n1436 = Multiply(x=w2003, y=60.0) -> (x*y=→"HP3 Flush Time (s)":dbl)
            n1437 = VISA Write(VISA resource name=w2020, write buffer=w2009) -> (VISA resource name out=w2008:refnum<visa-resource-name>)  [unwired: 1 in, 2 out]
            n1438 = Concatenate Strings("cvolume" ("string"), "\r") -> (w2007:string)
            n1439 = VISA Write(VISA resource name=w2008, write buffer=w2007) -> (VISA resource name out=w2018:refnum<visa-resource-name>)  [unwired: 1 in, 2 out]
            n1440 = Concatenate Strings("irun" ("string"), "\r") -> (w2016:string)
            n1441 = VISA Write(VISA resource name=w2018, write buffer=w2016) -> ()  [unwired: 1 in, 3 out]
          }
          frame #1 {
            "Flushing P3" <- TRUE ("Flushing P3")
          }
        }
      }
      event "Flush Pump 1": Value Change {
        n1442 = event-data() -> ()  [unwired: 7 out]
        n1443 = flat-sequence {
          tunnel: [w2038] -> w2028
          tunnel: w2027 -> [w2031]
          tunnel: w2028 -> [_]
          frame #0 {
            # "set paramaters (rate, volume) for flush, clear volume"
            n1444 = local write "Inject Pump 1"(TRUE ("Inject Pump 1")) -> ()
            n1445 = Number To Decimal String(number="Flush rate (uL/m) P1") -> (decimal integer string=w2054:string)  [unwired: 1 in]
            n1446 = Concatenate Strings("irate  " ("string"), w2054, " u/m" ("string"), "\r") -> (w2056:string)
            n1447 = VISA Write(VISA resource name=w2031, write buffer=w2056) -> (VISA resource name out=w2052:refnum<visa-resource-name>)  [unwired: 1 in, 2 out]
            n1448 = Reciprocal(x="Flush rate (uL/m) P1") -> (1/x=w2035:dbl)
            n1449 = Number To Decimal String(number="Volume (uL) P1") -> (decimal integer string=w2043:string)  [unwired: 1 in]
            n1450 = Multiply(x="Volume (uL) P1", y=w2035) -> (x*y=w2034:dbl)
            n1451 = Concatenate Strings("tvolume  " ("string"), w2043, " u" ("string"), "\r") -> (w2041:string)
            n1452 = Multiply(x=w2034, y=60.0) -> (x*y=→"HP1 Flush Time (s)":dbl)
            n1453 = VISA Write(VISA resource name=w2052, write buffer=w2041) -> (VISA resource name out=w2040:refnum<visa-resource-name>)  [unwired: 1 in, 2 out]
            n1454 = Concatenate Strings("cvolume" ("string"), "\r") -> (w2039:string)
            n1455 = VISA Write(VISA resource name=w2040, write buffer=w2039) -> (VISA resource name out=w2050:refnum<visa-resource-name>)  [unwired: 1 in, 2 out]
            n1456 = Concatenate Strings("irun" ("string"), "\r") -> (w2048:string)
            n1457 = VISA Write(VISA resource name=w2050, write buffer=w2048) -> (VISA resource name out=w2038:refnum<visa-resource-name>)  [unwired: 1 in, 2 out]
          }
          frame #1 {
            "Flushing P1" <- TRUE ("Flushing P3")
          }
        }
      }
      event "Clear Volume": Value Change {
        n1458 = event-data() -> ()  [unwired: 7 out]
        n1459 = Number To Decimal String(number="Normal volume (mL)") -> (decimal integer string=w2063:string)  [unwired: 1 in]
        n1460 = Concatenate Strings("tvolume " ("string"), w2063, " u" ("string"), "\r") -> (w2060:string)
        n1461 = VISA Write(VISA resource name=w2066, write buffer=w2060) -> (VISA resource name out=w2059:refnum<visa-resource-name>)  [unwired: 1 in, 2 out]
        n1462 = local write "Clear Volume"(FALSE ("Clear Volume")) -> ()
        n1463 = Concatenate Strings("cvolume" ("string"), "\r") -> (w2068:string)
        n1464 = VISA Write(VISA resource name=w2059, write buffer=w2068) -> ()  [unwired: 1 in, 3 out]
      }
      event "Clear Volume P3": Value Change {
        n1465 = event-data() -> ()  [unwired: 7 out]
        n1466 = Concatenate Strings("cvolume" ("string"), "\r") -> (w2074:string)
        n1467 = VISA Write(VISA resource name=w2073, write buffer=w2074) -> ()  [unwired: 1 in, 3 out]
        n1468 = local write "Clear Volume P3"(FALSE ("Clear Volume P3")) -> ()
      }
      event "Clear Volume P1": Value Change {
        n1469 = event-data() -> ()  [unwired: 7 out]
        n1470 = Concatenate Strings("cvolume" ("string"), "\r") -> (w2079:string)
        n1471 = local write "Clear Volume P1"(FALSE ("Clear Volume P1")) -> ()
        n1472 = VISA Write(VISA resource name=w2078, write buffer=w2079) -> ()  [unwired: 1 in, 3 out]
      }
      event "Display On P3": Value Change {
        n1473 = event-data() -> ()  [unwired: 7 out]
        n1474 = Select(t="dim 100", s="Display On P3", f="dim 0") -> (s? t:f=w2085:string)
        n1475 = Concatenate Strings(w2085, "\r") -> (w2087:string)
        n1476 = VISA Write(VISA resource name=w2082, write buffer=w2087) -> ()  [unwired: 1 in, 3 out]
      }
      event "Display On P1": Value Change {
        n1477 = event-data() -> ()  [unwired: 7 out]
        n1478 = Select(t="dim 100", s="Display On P1", f="dim 0") -> (s? t:f=w2092:string)
        n1479 = Concatenate Strings(w2092, "\r") -> (w2094:string)
        n1480 = VISA Write(VISA resource name=w2089, write buffer=w2094) -> ()  [unwired: 1 in, 3 out]
      }
      event "Retract Pump 3": Value Change {
        n1481 = event-data() -> ()  [unwired: 7 out]
        n1482 = local write "Retract Pump 3"(FALSE ("Retract Pump 3")) -> ()
        n1483 = case shown="True" "Retract Pump 3" {
          tunnel: w2096 -> [_ w2099]
          frame False {
          }
          frame True {
            n1484 = Number To Decimal String(number="Retract Rate (mL/m)") -> (decimal integer string=w2117:string)  [unwired: 1 in]
            n1485 = Concatenate Strings("wrate  " ("string"), w2117, " u/m" ("string"), "\r") -> (w2119:string)
            n1486 = VISA Write(VISA resource name=w2099, write buffer=w2119) -> (VISA resource name out=w2110:refnum<visa-resource-name>)  [unwired: 1 in, 2 out]
            n1487 = Number To Decimal String(number="Retract Vol 3 (uL)") -> (decimal integer string=w2112:string)  [unwired: 1 in]
            n1488 = Concatenate Strings("tvolume  " ("string"), w2112, " u" ("string"), "\r") -> (w2109:string)
            n1489 = VISA Write(VISA resource name=w2110, write buffer=w2109) -> (VISA resource name out=w2105:refnum<visa-resource-name>)  [unwired: 1 in, 2 out]
            n1490 = Concatenate Strings("cvolume" ("string"), "\r") -> (w2106:string)
            n1491 = VISA Write(VISA resource name=w2105, write buffer=w2106) -> (VISA resource name out=w2100:refnum<visa-resource-name>)  [unwired: 1 in, 2 out]
            n1492 = Concatenate Strings("wrun" ("string"), "\r") -> (w2101:string)
            n1493 = VISA Write(VISA resource name=w2100, write buffer=w2101) -> ()  [unwired: 1 in, 3 out]
          }
        }
      }
      event "Retract Pump 1": Value Change {
        n1494 = event-data() -> ()  [unwired: 7 out]
        n1495 = local write "Retract Pump 1"(FALSE ("Retract Pump 1")) -> ()
        n1496 = case shown="True" "Retract Pump 1" {
          tunnel: w2121 -> [_ w2126]
          frame False {
          }
          frame True {
            n1497 = local read "Retract Rate (mL/m)"() -> (w2124:dbl)
            n1498 = Number To Decimal String(number=w2124) -> (decimal integer string=w2142:string)  [unwired: 1 in]
            n1499 = Concatenate Strings("wrate  " ("string"), w2142, " u/m" ("string"), "\r") -> (w2144:string)
            n1500 = VISA Write(VISA resource name=w2126, write buffer=w2144) -> (VISA resource name out=w2136:refnum<visa-resource-name>)  [unwired: 1 in, 2 out]
            n1501 = Number To Decimal String(number="Retract Vol 1 (uL)") -> (decimal integer string=w2138:string)  [unwired: 1 in]
            n1502 = Concatenate Strings("tvolume  " ("string"), w2138, " u" ("string"), "\r") -> (w2135:string)
            n1503 = VISA Write(VISA resource name=w2136, write buffer=w2135) -> (VISA resource name out=w2132:refnum<visa-resource-name>)  [unwired: 1 in, 2 out]
            n1504 = Concatenate Strings("cvolume" ("string"), "\r") -> (w2133:string)
            n1505 = VISA Write(VISA resource name=w2132, write buffer=w2133) -> (VISA resource name out=w2127:refnum<visa-resource-name>)  [unwired: 1 in, 2 out]
            n1506 = Concatenate Strings("wrun" ("string"), "\r") -> (w2128:string)
            n1507 = VISA Write(VISA resource name=w2127, write buffer=w2128) -> ()  [unwired: 1 in, 3 out]
          }
        }
      }
      event "Flip Green Filter": Value Change {
        n1508 = event-data() -> ()  [unwired: 7 out]
        n1509 = Not(x="Flip Green Filter") -> (.not. x?=w2146:bool)
        n1510 = local write "Flip Green Filter"(w2146) -> ()
        n1511 = flat-sequence {
          tunnel: w2154 -> [w2159]
          tunnel: w2153 -> [w2158]
          tunnel: [w2156] -> w2151
          tunnel: [w2155] -> w2150
          tunnel: [w2161] -> w2149
          tunnel: w2151 -> [w2161]
          tunnel: [w2160] -> w2148
          tunnel: w2150 -> [w2160]
          tunnel: w2149 -> [w2165]
          tunnel: w2148 -> [w2164]
          tunnel: [w2163] -> w2152
          frame #0 {
            n1512 = xnode "Read/Write Control"("FPGA VI Reference In"=w2159, "error in"=w2158, "Green Filter Flipper"=TRUE) -> ("FPGA VI Reference Out"=w2156:T19, "error out"=w2155:errorcluster)
          }
          frame #1 {
            n1513 = Wait (ms)(milliseconds to wait=u32 100) -> ()  [unwired: 1 out]
          }
          frame #2 {
            n1514 = xnode "Read/Write Control"("FPGA VI Reference In"=w2165, "error in"=w2164, "Green Filter Flipper"=FALSE) -> ("error out"=w2163:errorcluster)  [unwired: 1 out]
          }
        }
      }
      event "Pump 1 contents", "Pump 3 contents": Value Change {
        n1515 = event-data() -> ()  [unwired: 7 out]
        n1516 = local read "Pump 1 contents"() -> (→"Pump 1 cont disp":string)
        n1517 = local read "Pump 3 contents"() -> (→"Pump 3 cont disp":string)
      }
      event "Reset Trap Pos. FB": Value Change {
        n1518 = event-data() -> ()  [unwired: 7 out]
        n1519 = xnode "Read/Write Control"("FPGA VI Reference In"=w2171, "error in"=w2170, "Trap Pos. FB Reset"="Reset Trap Pos. FB") -> ()  [unwired: 2 out]
      }
      event "Rem fb disp offset": Value Change {
        n1520 = event-data() -> ()  [unwired: 7 out]
        n1521 = local write "Rem fb disp offset"(FALSE ("Rem fb disp offset")) -> ()
        n1522 = local read "Mean T1 Position (nm)"() -> (w2173:dbl)
        n1523 = local read "FB Trap Pos Offset"() -> (w2174:dbl)
        n1524 = Subtract(x=w2174, y=w2173) -> (x-y=w2172:dbl)
        n1525 = local write "FB Trap Pos Offset"(w2172) -> ()
      }
      event "Threshold (nm)": Value Change {
        n1526 = event-data() -> ()  [unwired: 7 out]
        n1527 = flat-sequence {
          tunnel: w2178 -> [w2186]
          tunnel: w2177 -> [w2185]
          tunnel: [w2179] -> w2176
          tunnel: w2176 -> [w2192]
          frame #0 {
            n1528 = xnode "Read/Write Control"("FPGA VI Reference In"=w2186, "error in"=w2185) -> ("FPGA VI Reference Out"=w2182:T19, "error out"=w2181:errorcluster, "FPGA TTrig Thresh"=w2183:i64)
            n1529 = local read "Threshold stored (nm)"() -> (w2191:dbl)
            n1530 = local read "Threshold (nm)"() -> (w2179:dbl)
            n1531 = local read "AOM X Cal (nm/MHz)"() -> (w2189:dbl)
            n1532 = Subtract(x=w2179, y=w2191) -> (x-y=w2190:dbl)
            n1533 = Divide(x=w2190, y=w2189) -> (x/y=w2187:dbl)
            n1534 = call "IR AOM freq to word.vi"("Frequency In (MHz)"=w2187) -> ("Frequency Word Out (double)"=w2188:dbl)
            n1535 = To Quad Integer(1:w2188) -> (0:w2184:i64)
            n1536 = Add(x=w2183, y=w2184) -> (x+y=w2180:i64)
            n1537 = xnode "Read/Write Control"("FPGA VI Reference In"=w2182, "error in"=w2181, "FPGA TTrig Thresh"=w2180) -> ()  [unwired: 2 out]
          }
          frame #1 {
            "Threshold stored (nm)" <- w2192
          }
        }
      }
      event "FB Trig Integrate": Value Change {
        n1538 = event-data() -> ()  [unwired: 7 out]
        n1539 = local read "FB Trig Integrate"() -> (w2194:u32)
        n1540 = xnode "Read/Write Control"("FPGA VI Reference In"=w2196, "error in"=w2195, "FB Trig Integrate"=w2194) -> ("error out"=w2193:errorcluster)  [unwired: 1 out]
      }
      event "11": Value Change {
        n1541 = event-data() -> ()  [unwired: 7 out]
        n1542 = local read "11"() -> (w2197:bool)
        n1543 = case shown="True" w2197 {
          frame False {
          }
          frame True {
            n1544 = local read "Messages"() -> (w2199:string)
            n1545 = call "Update messages.vi"("Message to add"="You kicked it up to 11!", "Old message string"=w2199) -> ("New message string"=w2200:string)
            n1546 = call <vilib>:"Beep.vi"() -> ()  [unwired: 12 in]
            n1547 = local write "Messages"(w2200) -> ()
          }
        }
      }
      event "Trap Pos. FB ON": Value Change {
        n1548 = event-data() -> ()  [unwired: 7 out]
        n1549 = xnode "Read/Write Control"("FPGA VI Reference In"=w2203, "error in"=w2202, "Force feedback"="Trap Pos. FB ON") -> ()  [unwired: 2 out]
      }
      event "Remove Action Offset": Value Change {
        n1550 = event-data() -> ()  [unwired: 7 out]
        n1551 = local write "Remove Action Offset"(FALSE ("Remove Action Offset")) -> ()
        n1552 = local read "Trap Pos. FB Mult Factor"() -> (w2208:i64)
        n1553 = local read "Trap Pos FB Action"() -> (w2206:i64)
        n1554 = local read "Trap Pos. FB Offset Factor"() -> (w2204:i64)
        n1555 = Multiply(x=w2208, y=w2206) -> (x*y=w2207:i64)
        n1556 = Add(x=w2207, y=w2204) -> (x+y=w2205:i64)
        n1557 = local write "Trap Pos. FB Offset Factor"(w2205) -> ()
        n1558 = xnode "Read/Write Control"("FPGA VI Reference In"=w2211, "error in"=w2210, "Trap Pos. FB Offset Factor"=w2205) -> ()  [unwired: 2 out]
      }
      event "Remove Offset to factor": Value Change {
        n1559 = event-data() -> ()  [unwired: 7 out]
        n1560 = local write "Remove Offset to factor"(FALSE ("Remove Action Offset")) -> ()
        n1561 = local read "Trap Pos. FB Mult Factor"() -> (w2223:i64)
        n1562 = local read "Trap Pos FB Action"() -> (w2221:i64)
        n1563 = local read "Trap Pos. FB Offset Factor"() -> (w2220:i64)
        n1564 = Multiply(x=w2223, y=w2221) -> (x*y=w2222:i64)
